vi "Variable global de carga.vi"() -> ()   [LabVIEW 2019]
uses:
  Control 2.ctl
  <vilib>/Plasmionique/MB Master/MB_Master_Serial/MB_Master_Serial.lvclass
  <vilib>/Plasmionique/MB Master/MB_ADU_Serial/MB_ADU_Serial.lvclass
  <vilib>/Plasmionique/MB Master/MB_ADU_RTU/MB_ADU_RTU.lvclass
panel:
  in  "Controllers Number":u16
  in  "Array CtrConn":bool[](array[boolean])=[FALSE, FALSE, TRUE, FALSE, TRUE]
  in  "Recipe Number":u16
  in  "Conn":bool
  in  "Array Ran?":bool[](array[boolean])=[FALSE, FALSE, FALSE, FALSE, FALSE]
  in  "Array Running":bool[](array[boolean])=[FALSE, FALSE, FALSE, FALSE, FALSE]
  out "Array End Time":string[](array[string])=["", "", "30/07/2025 14:09:38", "", "30/07/2025 14:09:50"]
  out "Array Init Time":string[](array[string])
  out "Array Serials":T1
  in  "Global Running":bool
  out "Recipe Table":string[][](table)
  out "Loading Text":string
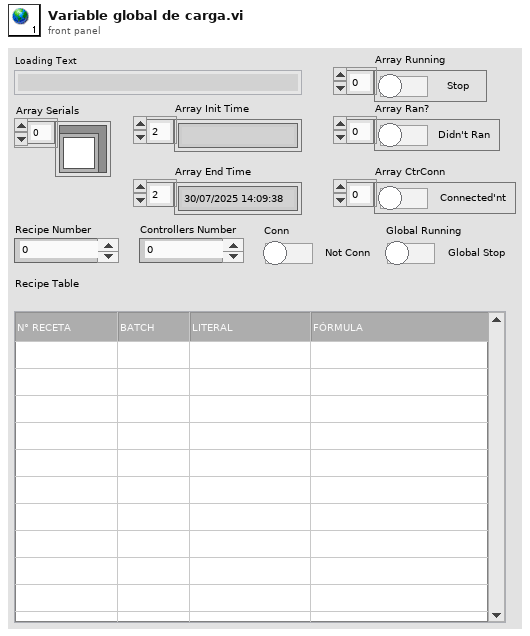
[diagram p1: front panel]
types:
  T1 = typedef "Control 2.ctl" = refnum<class "MB_Master_Serial.lvclass">[]
diagram:
